vi "localVar.vi"() -> ()   [LabVIEW 2019]
panel:
  in  "stop":bool
  out "Waveform Chart 2":dbl(graph)
  out "Waveform Chart":dbl(graph)
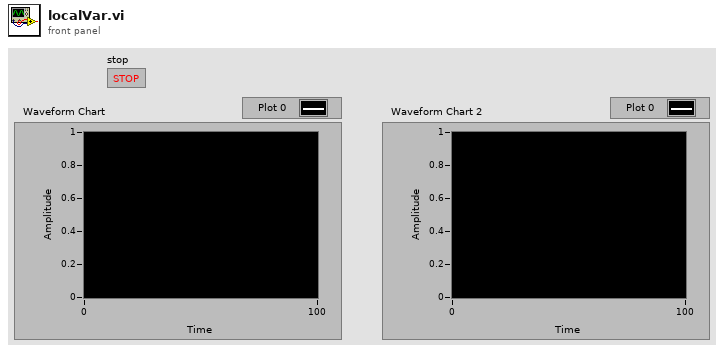
[diagram p1: front panel]
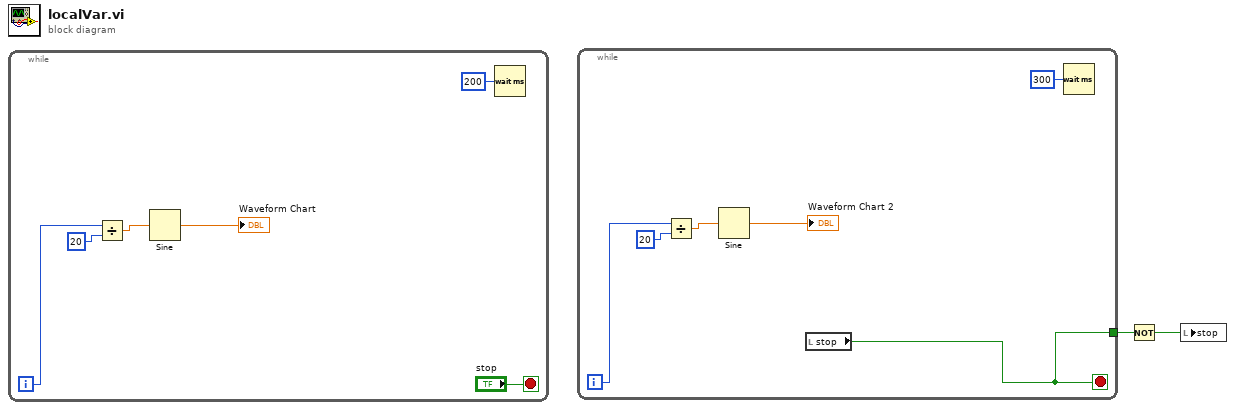
[diagram p0: block diagram]
diagram:
  n1 = while {
    i -> [w8]
    stop <- "stop" stop-if-true
    n2 = Divide(x=w8, y=20) -> (x/y=w6:dbl)
    n3 = Sine(x=w6) -> (sin(x)=→"Waveform Chart":dbl)
    n4 = Wait (ms)(milliseconds to wait=u32 200) -> ()  [unwired: 1 out]
  }
  n5 = while {
    tunnel: [w9] -> w2
    i -> [w14]
    stop <- w9 stop-if-true
    n6 = Divide(x=w14, y=20) -> (x/y=w12:dbl)
    n7 = Sine(x=w12) -> (sin(x)=→"Waveform Chart 2":dbl)
    n8 = local read "stop"() -> (w9:bool)
    n9 = Wait (ms)(milliseconds to wait=u32 300) -> ()  [unwired: 1 out]
  }
  n10 = Not(x=w2) -> (.not. x?=w1:bool)
  n11 = local write "stop"(w1) -> ()
